vi "set array elements (dbl 2d).vi"(0 "array in":dbl[][](array[numeric]), 5 "start 1":i32, 7 "end 1":i32=-1, 9 "start 2":i32, 11 "end 2":i32=-1, 12 "val":dbl) -> (4 "array out":dbl[][](array[numeric]))   [LabVIEW 2012, in "common.lvlib"]
uses:
  common.lvlib
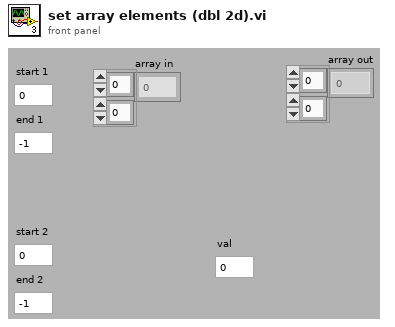
[diagram p1: front panel]
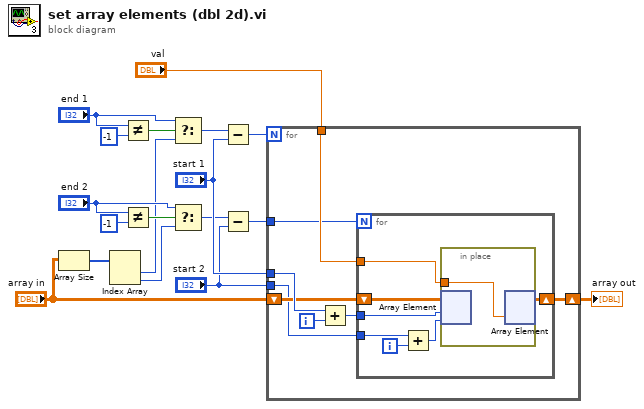
[diagram p0: block diagram]
diagram:
  n1 = Array Size(array="array in") -> (size(s)=w11:i32[])
  n2 = Index Array(array=w11) -> (element #1=w2:i32, element #2=w1:i32)  [unwired: 2 in]
  n3 = Not Equal?(x="end 1", y=-1 ("x")) -> (x != y?=w10:bool)
  n4 = Not Equal?(x="end 2", y=-1 ("x")) -> (x != y?=w6:bool)
  n5 = Select(t="end 1", s=w10, f=w2) -> (s? t:f=w3:i32)
  n6 = Select(t="end 2", s=w6, f=w1) -> (s? t:f=w4:i32)
  n7 = Subtract(x=w3, y="start 1") -> (x-y=w18:i32)
  n8 = Subtract(x=w4, y="start 2") -> (x-y=w14:i32)
  n9 = for {
    N: w18 -> [_]
    tunnel: "start 1" -> [w26]
    shift-right: [w21] -> w16
    shift-left: "array in" -> [w24]
    tunnel: "val" -> [w22]
    tunnel: w14 -> [w20]
    tunnel: "start 2" -> [w19]
    i -> [w25]
    n10 = Add(x=w26, y=w25) -> (x+y=w23:i32)
    n11 = for {
      N: w20 -> [_]
      tunnel: w23 -> [w32]
      tunnel: w22 -> [w31]
      tunnel: w19 -> [w28]
      shift-right: [w30] -> w21
      shift-left: w24 -> [w33]
      i -> [w29]
      n12 = Add(x=w28, y=w29) -> (x+y=w27:i32)
      n13 = in-place {
        in-place-border: w31 -> [w34]
        n14 = in-place-array #1(w33, w32, w27) -> ()  [unwired: 1 out]
        n15 = in-place-array #1(w34) -> (w30:dbl[][])  [unwired: 2 out]
      }
    }
  }
  "array out" <- w16
